vi "rad_Detect NIAuth.vi"(8 "error in (no error)":errorcluster, 11 "Session in":refnum<k21>) -> (0 "error out":errorcluster, 2 "Post-deployment access":T1, 3 "Session out":refnum<k21>)   [LabVIEW 2023]
uses:
  Targets/TypeDefs/rad_Initialize Access Types.ctl
  <vilib>/nisyscfg/Get Installed Components.vi
  <vilib>/nisyscfg/nisyscfg.lvlib
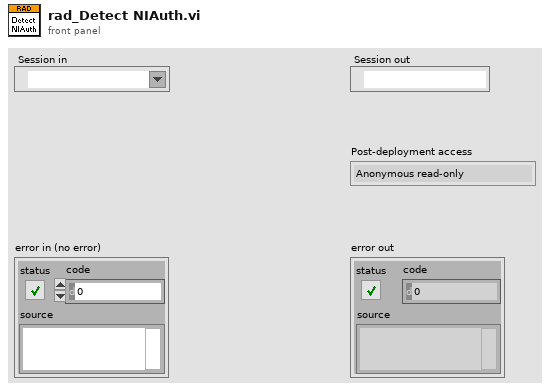
[diagram p1: front panel]
types:
  T1 = typedef "rad_Initialize Access Types.ctl" = enum16{"Anonymous read-only", "Admin unless unlocked", "Admin always"}
  T2 = typedef "nisyscfg.lvlib/Software 1.2.ctl" = cluster{"title":string, "description":string, "ID":string, "version":string, "component type":T3}
  T3 = typedef "nisyscfg.lvlib/Component Type.ctl" = u32
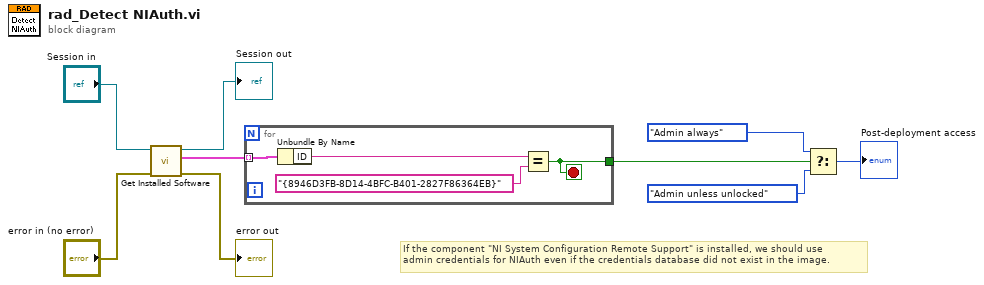
[diagram p0: block diagram]
diagram:
  # "If the component \"NI System Configuration Remote Support\" is installed, we should use\nadmin credentials for NIAuth even if the credentials database did not exist in the image."
  n1 = call-poly <vilib>:"Get Installed Software.vi"("error in (no error)"="error in (no error)", "Session in"="Session in") -> ("error out"=→"error out":errorcluster, "Software Components"=w8:T2[], "Session out"=→"Session out":refnum<k21>)  [unwired: 7 in]
  n2 = for {
    tunnel: w8 -> [w13] mode=indexing
    tunnel: [w10] -> w4
    stop <- w10 stop-if-true
    n3 = Unbundle By Name(w13) -> ("ID"=w12:string)
    n4 = Equal?(x=w12, y="{8946D3FB-8D14-4BFC-B401-2827F86364EB}") -> (x = y?=w10:bool)
  }
  n5 = Select(t=rad_Initialize_Access_Types."Admin always" ("Post-deployment access"), s=w4, f=rad_Initialize_Access_Types."Admin unless unlocked" ("Post-deployment access")) -> (s? t:f=→"Post-deployment access":T1)
